vi "Jog Axis.vi"(4 "error in (no error)":errorcluster, 5 "Jog Speed":sgl, 6 "Axis In":i16, 7 "Controller Reference":refnum<k7>) -> (0 "error out":errorcluster, 2 "Axis Out":i16, 3 "Controller Reference out":refnum<k7>)   [LabVIEW 2015]
doc: "Starts the specified axis 'Jogging' at the input Speed. A 'Jogging' axis will continue moving until a Stop command is sent. Negative values for Jog Speed will cause movement in the opposite direction."
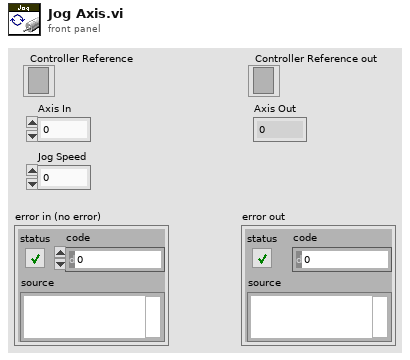
[diagram p1: front panel]
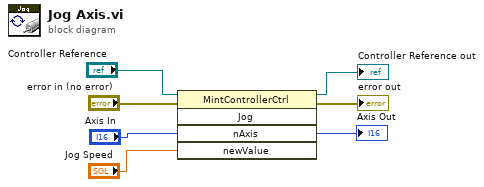
[diagram p0: block diagram]
diagram:
  n1 = invoke class="MintControllerCtrl" method="Jog"(reference="Controller Reference", error in="error in (no error)", "nAxis"="Axis In", "newValue"="Jog Speed") -> (reference out=→"Controller Reference out":refnum<k7>, error out=→"error out":errorcluster, "nAxis"=→"Axis Out":i16)  [unwired: 1 in, 2 out]
